vi "Set COM Output Scan Direction.vi"(8 "Error In":errorcluster, 10 "COM Direction":enum8{"COM0 -> COM[N-1]", "COM[N-1] -> COM0"}(ring), 11 "LINX Resource":T1) -> (0 "Error Out":errorcluster, 3 "LINX Resource":T1)   [LabVIEW 2013, in "LVH-LINX.lvlib" / "SSD1306.lvlib"]
doc: "Set the SSD1306 COM scan direction."
uses:
  <vilib>/LabVIEW Hacker/LINX/Public/Sensors/Display/SSD1306/SSD1306.lvlib
  <vilib>/LabVIEW Hacker/LINX/Private/Type Defs/LINX Ref.ctl
  <vilib>/LabVIEW Hacker/LINX/Private/Type Defs/Platform.ctl
  <vilib>/LabVIEW Hacker/LINX/Private/Type Defs/Interface.ctl
  <vilib>/LabVIEW Hacker/LINX/Private/Device/Type Defs/LINX Device Config.ctl
  <vilib>/LabVIEW Hacker/LINX/Private/Device/Type Defs/TCP Config.ctl
  <vilib>/LabVIEW Hacker/LINX/Private/Type Defs/Device Family.ctl
  <vilib>/LabVIEW Hacker/LINX/Public/Sensors/Display/SSD1306/Private/SSD1306 FGV State.ctl
  <vilib>/LabVIEW Hacker/LINX/Public/Peripherals/Digital/Digital Write 1 Chan.vi
  <vilib>/LabVIEW Hacker/LINX/LVH-LINX.lvlib
  <vilib>/LabVIEW Hacker/LINX/Private/Device/Device.lvlib
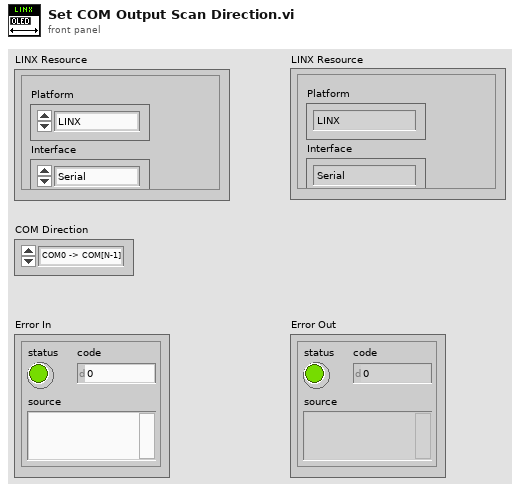
[diagram p1: front panel]
types:
  T1 = typedef "LVH-LINX.lvlib/LINX Ref.ctl" = cluster{"Platform":T2, "Interface":T3, "LINX Device Config":T4}
  T2 = typedef "LVH-LINX.lvlib/Platform.ctl" = enum16{"LINX", "myRIO"}
  T3 = typedef "LVH-LINX.lvlib/Interface.ctl" = enum16{"Serial", "TCP"}
  T4 = typedef "LVH-LINX.lvlib/Device.lvlib/LINX Device Config.ctl" = cluster{"Interface":T3, "COM Port":refnum<visa-resource-name>, "TCP Configuration":T5, "Device Family":T6, "Device ID":u8, "Device Name":string, "TCP Ref":refnum<k5>}
  T5 = typedef "LVH-LINX.lvlib/Device.lvlib/TCP Config.ctl" = cluster{"IP Address":string, "Port":u16}
  T6 = typedef "LVH-LINX.lvlib/Device Family.ctl" = enum8{"National Instruments", "Digilent", "Arduino"}
  T7 = typedef "LVH-LINX.lvlib/SSD1306.lvlib/SSD1306 FGV State.ctl" = enum16{"Init", "Set", "Get"}
  T8 = typedef "LVH-LINX.lvlib/SSD1306.lvlib/SSD1306 Config.ctl" = cluster{"SPI Channel (0)":u8, "VDD Channel":u8, "VBAT Channel":u8, "RESET Channel":u8, "DC Channel":u8, "SPI CS (3)":u8}
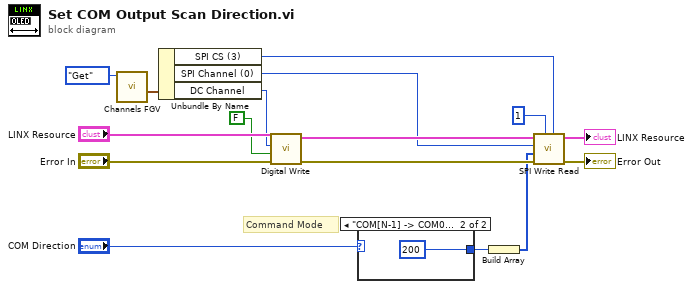
[diagram p0: block diagram]
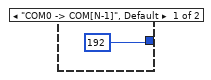
[diagram p2: hidden frame]
diagram:
  # "Command Mode"
  n1 = call <vilib>:"Channels FGV.vi"("SSD1306 FGV State"=SSD1306_FGV_State."Get") -> ("SSD1306 Channels"=w13:T8)  [unwired: 10 in]
  n2 = Unbundle By Name(w13) -> ("SPI CS (3)"=w1:u8, "SPI Channel (0)"=w8:u8, "DC Channel"=w12:u8)
  n3 = call-poly <vilib>:"Digital Write.vi"("Error In"="Error In", "Output Value"=FALSE, "DO Channel"=w12, "LINX Resource"="LINX Resource") -> ("Error Out"=w9:errorcluster, "LINX Resource"=w10:T1)  [unwired: 6 in]
  n4 = case shown="\"COM[N-1] -> COM0\"" "COM Direction" {
    tunnel: [u8 192 ("SPI Frame Size") u8 200 ("SPI Frame Size")] -> w3
    frame "COM0 -> COM[N-1]", Default {
    }
    frame "COM[N-1] -> COM0" {
    }
  }
  n5 = Build Array(w3) -> (w2:u8[])
  n6 = call <vilib>:"SPI Write Read.vi"("CS Pin (10)"=w1, "SPI Frame Size"=u8 1, "Error In"=w9, "Data"=w2, "SPI Channel (0)"=w8, "LINX Resource"=w10) -> ("Error Out"=→"Error Out":errorcluster, "LINX Resource"=→"LINX Resource":T1)  [unwired: 3 in, 1 out]
